vi "autoshutdown_IPS.vi"() -> ()   [LabVIEW 2016]
uses:
  Equipment/Oxford Software/Oxsoft/RAMP.LLB/RampHState.ctl
  Equipment/Oxford Software/Oxsoft/RAMP.LLB/RampTState.ctl
  Global Variables/Data_Display_global.vi
  Instrument_Setup.vi
panel:
  in  "Ramp Parameters":T1 {"Sweep rate" format="%.2f"; "Field required:" format="%.2f"}
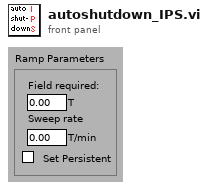
[diagram p1: front panel]
types:
  T1 = cluster{"Field required:":dbl[unit], "Sweep rate":dbl[unit], "Set Persistent":bool}
  T2 = typedef "RampHState.ctl" = enum16{"START", "RUN"}
  T3 = typedef "RampTState.ctl" = enum16{"START", "RUN"}
  T4 = typedef "PSIO.ctl" = cluster{"Address":T5, "Version":enum16{"PS", "IPS"}}
  T5 = typedef "OxfordAddress.ctl" = cluster{"Com Port":i32, "ISOBUS Address":i32, "GPIB Address":i16, "Communication":enum16{"RS232", "ISOBUS", "GPIB", "Gateway"}}
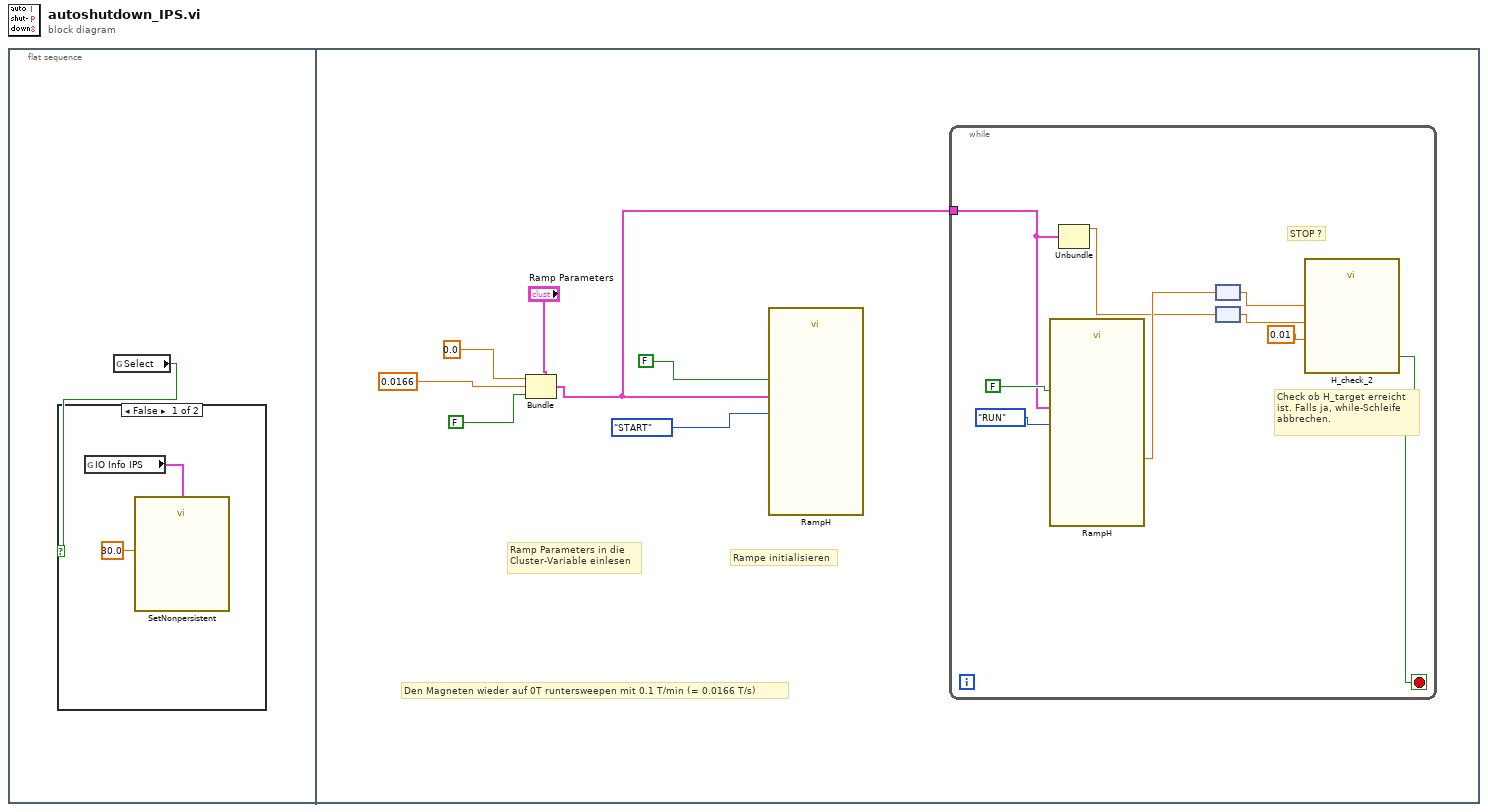
[diagram p0: block diagram]
diagram:
  n1 = flat-sequence {
    frame #0 {
      n2 = global read "Data_Display_global.vi" "Select"() -> (w1:bool)
      n3 = case shown="False" w1 {
        frame False {
          n4 = global read "Instrument_Setup.vi" "IO Info IPS"() -> (w3:T4)
          n5 = call "SetNonpersistent.vi"("Switch Heater Dwell Time"=dbl[unit] 30.0, "IO Info"=w3) -> ()  [unwired: 2 out]
        }
        frame True {
        }
      }
    }
    frame #1 {
      # "Den Magneten wieder auf 0T runtersweepen mit 0.1 T/min (= 0.0166 T/s)"
      # "Rampe initialisieren"
      # "Ramp Parameters in die \nCluster-Variable einlesen"
      n6 = Bundle(cluster="Ramp Parameters", "Field required:"=dbl[unit] 0.0, "Sweep rate"=dbl[unit] 0.0166, "Set Persistent"=FALSE) -> (w4:T1)
      n7 = call "RampH.vi"("Ramp Parameters"=w4, "JustReadField"=FALSE ("JustReadTemperature"), "RampHState"=RampHState."START") -> ()  [unwired: 4 in, 5 out]
      n8 = while {
        tunnel: w4 -> [w13]
        stop <- w12 stop-if-true
        # "Check ob H_target erreicht\nist. Falls ja, while-Schleife\nabbrechen."
        # "STOP ?"
        n9 = call "RampH.vi"("Ramp Parameters"=w13, "JustReadField"=FALSE ("JustReadTemperature"), "RampHState"=RampTState."RUN" ("RampTState")) -> ("Effective field"=w17:dbl[unit])  [unwired: 4 in, 4 out]
        n10 = Unbundle(w13) -> ("Field required:"=w16:dbl[unit])  [unwired: 2 out]
        n11 = node(w17) -> (w15:dbl)
        n12 = node(w16) -> (w14:dbl)
        n13 = call "H_check_2.vi"("Sweep\nTolerance %"=0.01 ("Sweep\nTolerance %"), "H_in"=w15, "H_target (K)"=w14) -> ("= H target"=w12:bool)  [unwired: 8 in]
      }
    }
  }
